vi "TMS burst generator (SubVI).vi"(3 "percent for random":dbl=20.0, 4 "nominal freq (Hz)":i32=20, 5 "H duration (ms)":i32=10, 6 "Total duration (ms)":i32=1000) -> (0 "Timing (ms)":i32[](array[numeric]), 1 "digital waveform":digitalwaveform(waveform), 2 "out":bool[](array[boolean]))   [LabVIEW 2011]
uses:
  <vilib>/Waveform/DWDTOps.llb/DWDT Boolean Array to Digital.vi
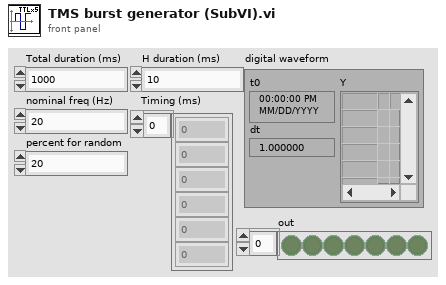
[diagram p1: front panel]
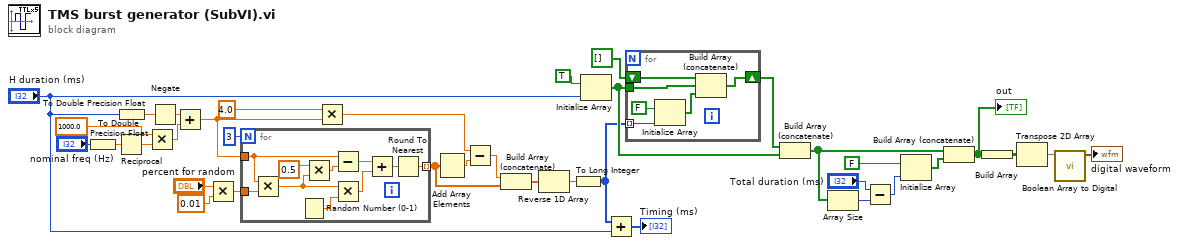
[diagram p0: block diagram]
diagram:
  n1 = To Double Precision Float(number="nominal freq (Hz)") -> (double precision float=w20:dbl)
  n2 = Reciprocal(x=w20) -> (1/x=w23:dbl)
  n3 = To Double Precision Float(number="H duration (ms)") -> (double precision float=w21:dbl)
  n4 = Multiply(x=1000.0, y=w23) -> (x*y=w26:dbl)
  n5 = Negate(x=w21) -> (-x=w25:dbl)
  n6 = Add(x=w25, y=w26) -> (x+y=w22:dbl)
  n7 = Multiply(x="percent for random", y=0.01) -> (x*y=w28:dbl)
  n8 = for {
    N: 3 -> [_]
    tunnel: w22 -> [w43]
    tunnel: w28 -> [w44]
    tunnel: [w45] -> w29 mode=indexing
    n9 = Multiply(x=w43, y=w44) -> (x*y=w39:dbl)
    n10 = Random Number (0-1)() -> (number: 0 to 1=w40:dbl)
    n11 = Multiply(x=0.5, y=w39) -> (x*y=w38:dbl)
    n12 = Subtract(x=w43, y=w38) -> (x-y=w42:dbl)
    n13 = Multiply(x=w39, y=w40) -> (x*y=w41:dbl)
    n14 = Add(x=w42, y=w41) -> (x+y=w46:dbl)
    n15 = Round To Nearest(number=w46) -> (nearest integer value=w45:dbl)
  }
  n16 = Multiply(x=4.0, y=w22) -> (x*y=w16:dbl)
  n17 = Add Array Elements(numeric array=w29) -> (sum=w19:dbl)
  n18 = Subtract(x=w16, y=w19) -> (x-y=w30:dbl)
  n19 = Build Array (concatenate)(w30, w29) -> (w31:dbl[])
  n20 = Reverse 1D Array(array=w31) -> (reversed array=w32:dbl[])
  n21 = To Long Integer(number=w32) -> (32bit integer=w2:i32[])
  n22 = Initialize Array(TRUE, "H duration (ms)") -> (w5:bool[])
  n23 = Add(x=w2, y="H duration (ms)") -> (x+y=→"Timing (ms)":i32[])
  n24 = for {
    tunnel: w2 -> [w52] mode=indexing
    shift-right: [w47] -> w13
    shift-left: bool[] [] -> [w48]
    tunnel: w5 -> [w51]
    n25 = Initialize Array(FALSE, w52) -> (w49:bool[])
    n26 = Build Array (concatenate)(w48, w51, w49) -> (w47:bool[])
  }
  n27 = Build Array (concatenate)(w13, w5) -> (w12:bool[])
  n28 = Array Size(array=w12) -> (size(s)=w10:i32)
  n29 = Subtract(x="Total duration (ms)", y=w10) -> (x-y=w8:i32)
  n30 = Initialize Array(FALSE, w8) -> (w7:bool[])
  n31 = Build Array (concatenate)(w12, w7) -> (w34:bool[])
  "out" <- w34
  n32 = Build Array(w34) -> (w35:bool[][])
  n33 = Transpose 2D Array(2D array=w35) -> (transposed array=w36:bool[][])
  n34 = call-poly <vilib>:"Boolean Array to Digital.vi"("boolean array"=w36) -> ("digital waveform"=→"digital waveform":digitalwaveform)  [unwired: 9 in, 1 out]
